vi "ReadDID.vi"(8 "error in (no error)":errorcluster, 10 "ID":u16, 11 "Connection Info":T1) -> (0 "error out":errorcluster, 3 "Connection Info":T1)   [LabVIEW 2015, in "Diagnostics Host Automation API.lvlib"]
uses:
  Diagnostics Host Automation API.lvlib
  <userlib>/STM/TCP/stm_TCP Connection Info.ctl
  <userlib>/STM/_SubVIs/stm_MetaDataElement.ctl
  <userlib>/STM/TCP/STM Write Message (TCP).vi
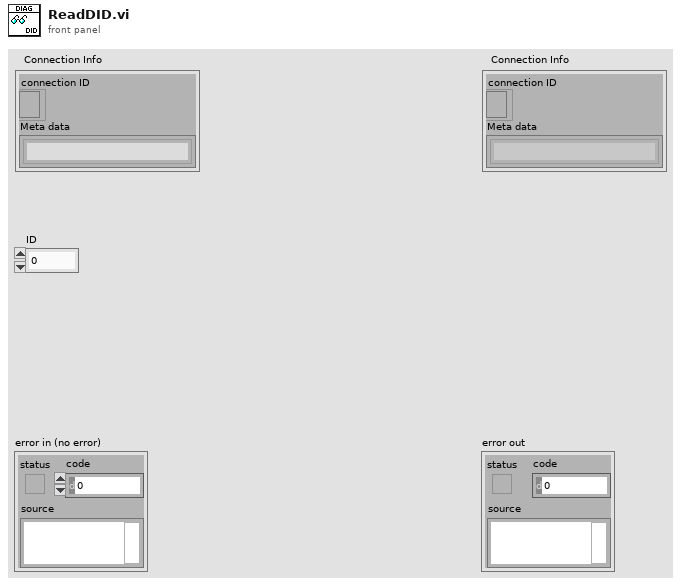
[diagram p1: front panel]
types:
  T1 = typedef "stm_TCP Connection Info.ctl" = cluster{"connection ID":refnum<k5>, "Meta data":T2[]}
  T2 = typedef "stm_MetaDataElement.ctl" = string
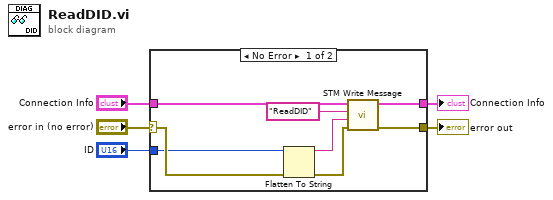
[diagram p0: block diagram]
diagram:
  n1 = case shown="No Error" "error in (no error)" {
    selector: "error in (no error)" -> [w8 w15]
    tunnel: "Connection Info" -> [w13 w14]
    tunnel: [w12 w14] -> w4
    tunnel: [w11 w15] -> w3
    tunnel: "ID" -> [w6 _]
    frame No Error {
      n2 = Flatten To String(anything=w6, error in (no error)=w8) -> (data string=w9:string, error out=w7:errorcluster)  [unwired: 2 in, 1 out]
      n3 = call-poly <userlib>:"STM Write Message.vi"("error in (no error)"=w7, "Data"=w9, "Name"="ReadDID", "Connection Info"=w13) -> ("error out"=w11:errorcluster, "Connection Info Out"=w12:T1)  [unwired: 6 in]
    }
    frame Error {
    }
  }
  "Connection Info" <- w4
  "error out" <- w3
